vi "spotfindsettings.vi"(7 "Enum":T3(ring), 9 "already x spots found":i16, 10 "first scan?":bool, 11 "notes 2":refnum<vi>) -> (0 "settings":string, 2 "spotfinding settings":T2={"show all"=FALSE, "threshold/morph"=FALSE, "particle filter"=FALSE, "spot marks"=FALSE, "close filter"=FALSE, "connectivity 4/8"=FALSE, "range"={"Lower value"=30.0, "Upper value"=30.0}, "PSF-size"=0, "Parameters"=[]} {"range"."Upper value" format="%.2f"; "range"."Lower value" format="%.2f"; "Parameters"."Upper Value" format="%.2f"; "Parameters"."Lower Value" format="%.2f"}, 4 "coordinates":i32[][](array[numeric]))   [LabVIEW 2009]
uses:
  spotfindersettings.ctl
panel:
  in  "range":cluster{"min.":i32, "max.":i32}={"min."=30, "max."=255}
  out "Number of Particles":i32
  in  "UPDATE":bool
  in  "Selection Values":T1(array[cluster]) {"Upper Value" format="%.2f"; "Lower Value" format="%.2f"}
  in  "scroll":u32 max=1
  in  "notes":string
  in  "spot marks":bool
  in  "particle filter":bool
  in  "threshold/morph":bool
  in  "show all":bool
  in  "PSF-size":i32=15
  in  "connectivity 4/8":bool
  in  "close filter":bool
  in  "add button":bool
  in  "delete button":bool
  in  "delete element":i32 min=0 max=0
  in  "stop":bool
  # "Selection Values"
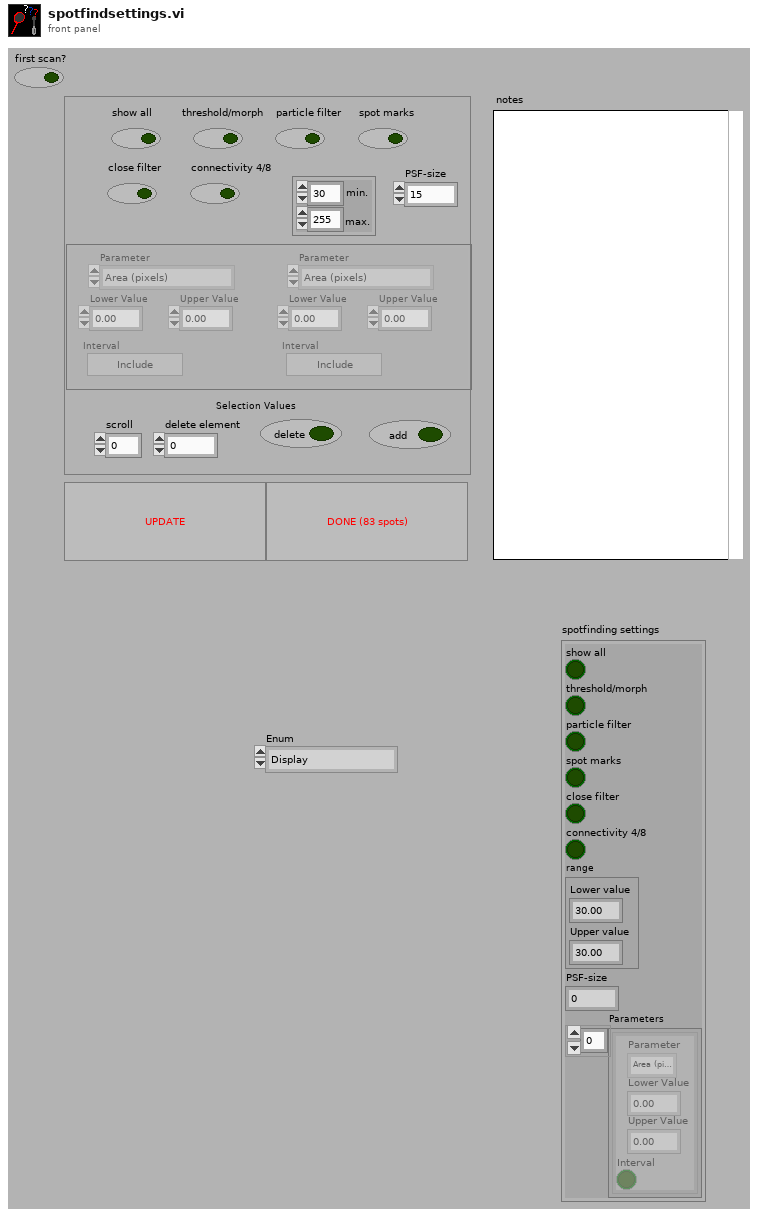
[diagram p1: front panel]
types:
  T1 = cluster{"Parameter":enum32{"Area (pixels)", "Area (calibrated)", "Number of holes", "Holes area (pixels)", "Total area (pixels)", "Scanned area (pixels)", "Ratio Area/Scanned area (%)", "Ratio Area/Total area (%)", "Center of mass (X)", "Center of mass (Y)", "Left column (X)", "Upper row (Y)", "Right column (X)", "Lower row (Y)", "Width (pixels)", "Height (pixels)", "Longest segment length", "Longest segment left column (X)", "Longest segment top row  (Y)", "Perimeter", "Holes perimeter", "SumX", "SumY", "SumXX", "SumYY", "SumXY", "Corrected projection X", "Corrected projection Y", "Moment of inertia Ixx", "Moment of inertia Iyy", "Moment of inertia Ixy", "Mean chord X", "Mean chord Y", "Max intercept", "Mean intercept perpendicular", "Particle orientation", "Equivalent ellipse minor axis", "Ellipse major axis", "Ellipse minor axis", "Ratio of equivalent ellipse axis", "Rectangle big side", "Rectangle small side", "Ratio of equivalent rectangle sides", "Elongation factor", "Compactness factor", "Heywood circularity factor", "Type factor", "Hydraulic radius", "Waddel disk diameter", "Diagonal"}, "Lower Value":sgl, "Upper Value":sgl, "Interval":bool}[]
  T2 = typedef "spotfindersettings.ctl" = cluster{"show all":bool, "threshold/morph":bool, "particle filter":bool, "spot marks":bool, "close filter":bool, "connectivity 4/8":bool, "range":cluster{"Lower value":sgl, "Upper value":sgl}, "PSF-size":i32, "Parameters":cluster{"Parameter":enum32{"Area (pixels)", "Area (calibrated)", "Number of holes", "Holes area (pixels)", "Total area (pixels)", "Scanned area (pixels)", "Ratio Area/Scanned area (%)", "Ratio Area/Total area (%)", "Center of mass (X)", "Center of mass (Y)", "Left column (X)", "Upper row (Y)", "Right column (X)", "Lower row (Y)", "Width (pixels)", "Height (pixels)", "Longest segment length", "Longest segment left column (X)", "Longest segment top row  (Y)", "Perimeter", "Holes perimeter", "SumX", "SumY", "SumXX", "SumYY", "SumXY", "Corrected projection X", "Corrected projection Y", "Moment of inertia Ixx", "Moment of inertia Iyy", "Moment of inertia Ixy", "Mean chord X", "Mean chord Y", "Max intercept", "Mean intercept perpendicular", "Particle orientation", "Equivalent ellipse minor axis", "Ellipse major axis", "Ellipse minor axis", "Ratio of equivalent ellipse axis", "Rectangle big side", "Rectangle small side", "Ratio of equivalent rectangle sides", "Elongation factor", "Compactness factor", "Heywood circularity factor", "Type factor", "Hydraulic radius", "Waddel disk diameter", "Diagonal"}, "Lower Value":sgl, "Upper Value":sgl, "Interval":bool}[]}
  T3 = enum16{"Display", "change", "get", "save", "create text", "load", "Get Refnum"}
  T4 = enum16{"Ini", "Get", "Set", "Refresh", "dump", "move", "name"}
  T5 = cluster{"show all":bool, "threshold/morph":bool, "particle filter":bool, "spot marks":bool, "close filter":bool, "connectivity 4/8":bool, "range":cluster{"Lower value":sgl, "Upper value":sgl}, "PSF-size":i32, "Parameters":cluster{"Parameter":enum32{"Area (pixels)", "Area (calibrated)", "Number of holes", "Holes area (pixels)", "Total area (pixels)", "Scanned area (pixels)", "Ratio Area/Scanned area (%)", "Ratio Area/Total area (%)", "Center of mass (X)", "Center of mass (Y)", "Left column (X)", "Upper row (Y)", "Right column (X)", "Lower row (Y)", "Width (pixels)", "Height (pixels)", "Longest segment length", "Longest segment left column (X)", "Longest segment top row  (Y)", "Perimeter", "Holes perimeter", "SumX", "SumY", "SumXX", "SumYY", "SumXY", "Corrected projection X", "Corrected projection Y", "Moment of inertia Ixx", "Moment of inertia Iyy", "Moment of inertia Ixy", "Mean chord X", "Mean chord Y", "Max intercept", "Mean intercept perpendicular", "Particle orientation", "Equivalent ellipse minor axis", "Ellipse major axis", "Ellipse minor axis", "Ratio of equivalent ellipse axis", "Rectangle big side", "Rectangle small side", "Ratio of equivalent rectangle sides", "Elongation factor", "Compactness factor", "Heywood circularity factor", "Type factor", "Hydraulic radius", "Waddel disk diameter", "Diagonal"}, "Lower Value":sgl, "Upper Value":sgl, "Interval":bool}[]}
  T6 = typedef "IMAQ Image.ctl" = refnum<image>
  T7 = enum32{"Area (pixels)", "Area (calibrated)", "Number of holes", "Holes area (pixels)", "Total area (pixels)", "Scanned area (pixels)", "Ratio Area/Scanned area (%)", "Ratio Area/Total area (%)", "Center of mass (X)", "Center of mass (Y)", "Left column (X)", "Upper row (Y)", "Right column (X)", "Lower row (Y)", "Width (pixels)", "Height (pixels)", "Longest segment length", "Longest segment left column (X)", "Longest segment top row  (Y)", "Perimeter", "Holes perimeter", "SumX", "SumY", "SumXX", "SumYY", "SumXY", "Corrected projection X", "Corrected projection Y", "Moment of inertia Ixx", "Moment of inertia Iyy", "Moment of inertia Ixy", "Mean chord X", "Mean chord Y", "Max intercept", "Mean intercept perpendicular", "Particle orientation", "Equivalent ellipse minor axis", "Ellipse major axis", "Ellipse minor axis", "Ratio of equivalent ellipse axis", "Rectangle big side", "Rectangle small side", "Ratio of equivalent rectangle sides", "Elongation factor", "Compactness factor", "Heywood circularity factor", "Type factor", "Hydraulic radius", "Waddel disk diameter", "Diagonal"}
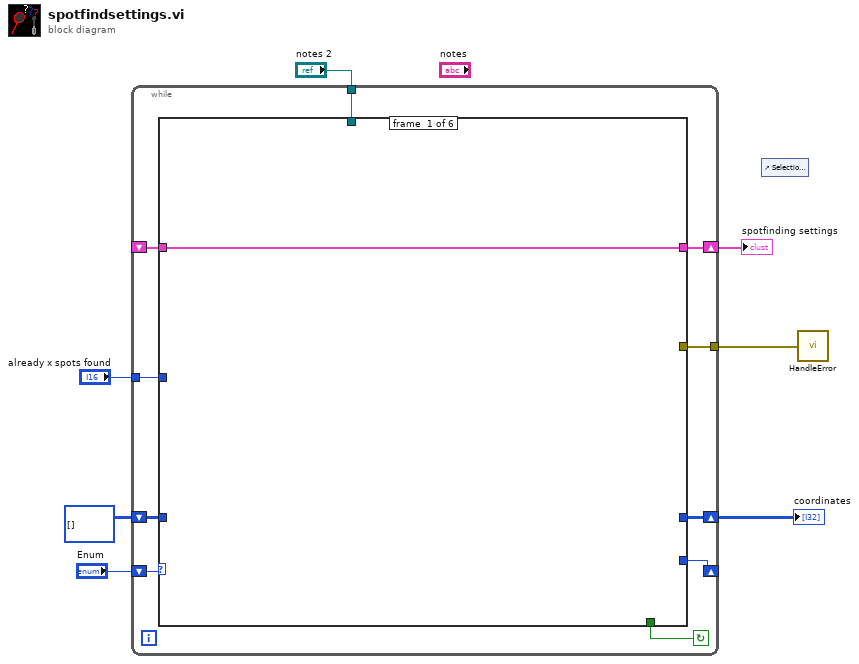
[diagram p0: block diagram]
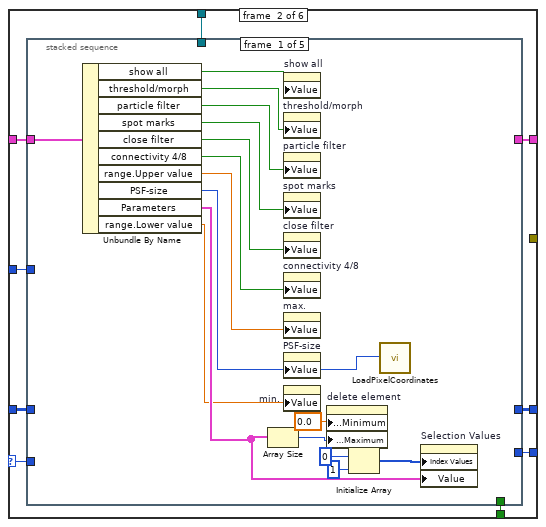
[diagram p2: hidden frame]
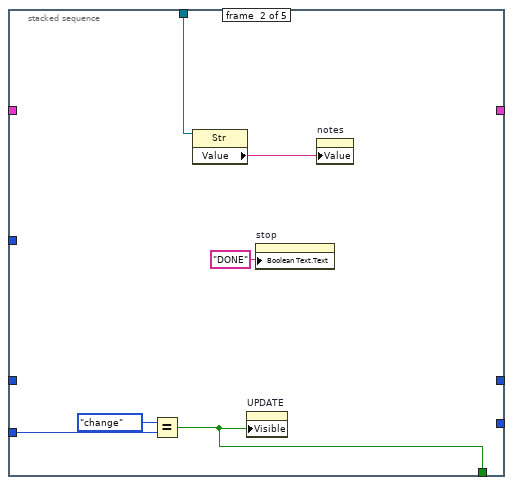
[diagram p3: hidden frame]
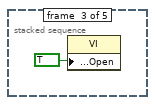
[diagram p4: hidden frame]
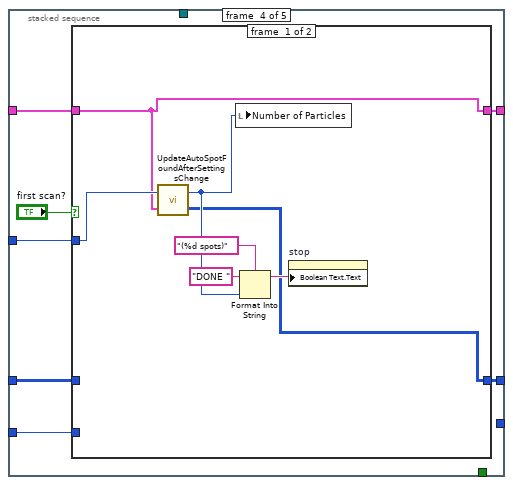
[diagram p5: hidden frame]
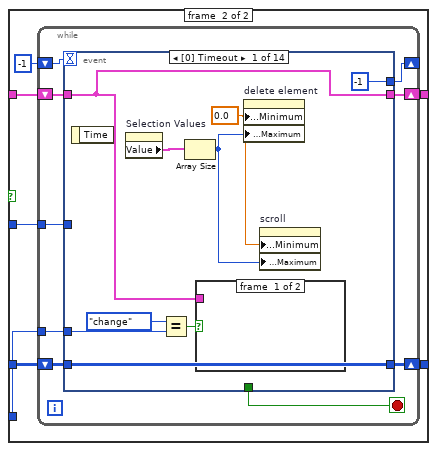
[diagram p6: hidden frame]
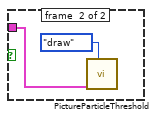
[diagram p7: hidden frame]
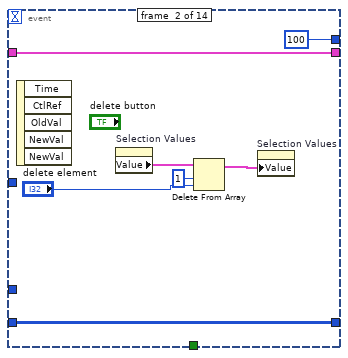
[diagram p8: hidden frame]
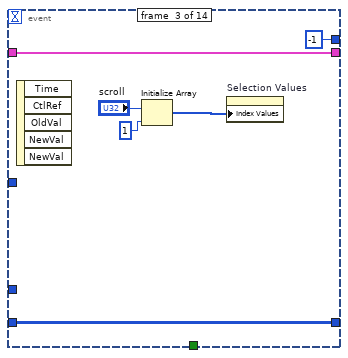
[diagram p9: hidden frame]
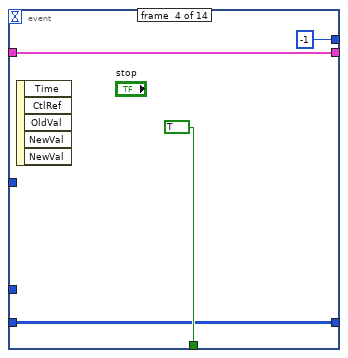
[diagram p10: hidden frame]
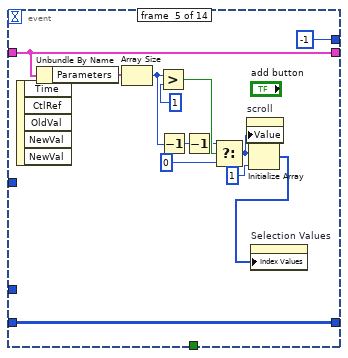
[diagram p11: hidden frame]
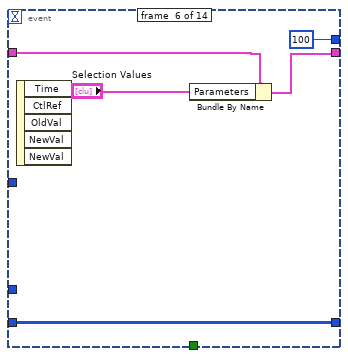
[diagram p12: hidden frame]
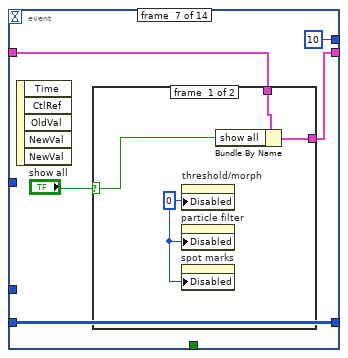
[diagram p13: hidden frame]
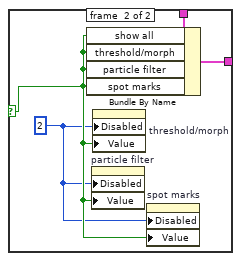
[diagram p14: hidden frame]
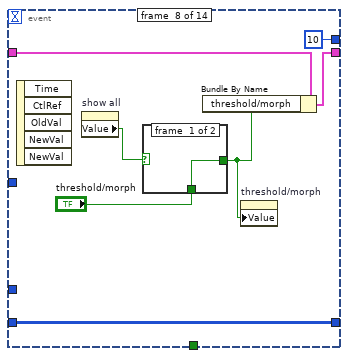
[diagram p15: hidden frame]
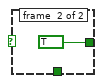
[diagram p16: hidden frame]
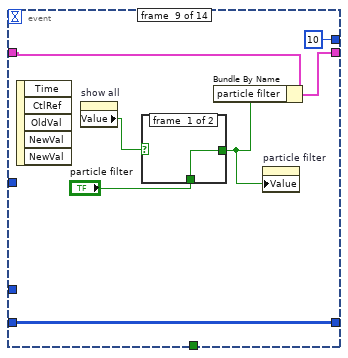
[diagram p17: hidden frame]
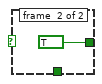
[diagram p18: hidden frame]
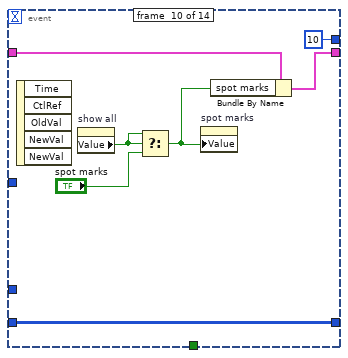
[diagram p19: hidden frame]
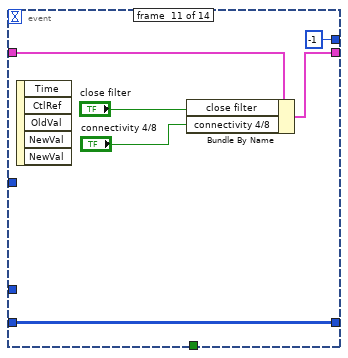
[diagram p20: hidden frame]
diagram:
  n1 = while {
    shift-right: [w8] -> w2
    shift-left: _ -> [w9]
    tunnel: [w17] -> w1
    tunnel: "notes 2" -> [w16]
    tunnel: "already x spots found" -> [w15]
    shift-right: [w12] -> _
    shift-left: "Enum" -> [w13]
    shift-right: [w10] -> w3
    shift-left: i32[][] [] ("coordinates") -> [w11]
    stop <- w14 continue-if-true
    n2 = case shown="\"Display\", \"change\"" w13 {
      selector: w13 -> [_ w21 _ _ _ _]
      tunnel: w9 -> [w18 w27 w206 w239 w245 _]
      tunnel: [_ _ _ _ w247 _] -> w17
      tunnel: w16 -> [_ w26 _ _ _ _]
      tunnel: w15 -> [_ w25 _ _ _ _]
      tunnel: [_ w24 _ _ _ _] -> w14
      tunnel: [_ w23 _ _ _ _] -> w12
      tunnel: [_ w22 w207 _ _ _] -> w10
      tunnel: w11 -> [_ w20 w207 _ _ _]
      tunnel: [w18 w19 w206 w240 w245 w252] -> w8
      frame #0 {
      }
      frame #1 {
        n3 = stacked-sequence {
          tunnel: w27 -> [w41 _ _ w57 _]
          tunnel: [_ _ _ w56 _] -> w19
          tunnel: w26 -> [_ w49 _ _ w203]
          tunnel: w25 -> [_ _ _ w55 _]
          tunnel: [_ w45 _ _ _] -> w24
          tunnel: [_ _ _ _ T3."create text" ("Enum")] -> w23
          tunnel: [_ _ _ w53 _] -> w22
          tunnel: w21 -> [_ w47 _ w54 _]
          tunnel: w20 -> [_ _ _ w52 _]
          frame #0 {
            n4 = Unbundle By Name(w41) -> ("show all"=w40:bool, "threshold/morph"=w39:bool, "particle filter"=w38:bool, "spot marks"=w37:bool, "close filter"=w36:bool, "connectivity 4/8"=w35:bool, "range.Upper value"=w34:sgl, "PSF-size"=w33:i32, "Parameters"=w29:T1, "range.Lower value"=w28:sgl)
            n5 = Array Size(array=w29) -> (size(s)=w42:i32)
            n6 = property on="show all" class="Bool (strict)"("Value"=w40) -> ()  [unwired: 2 in, 2 out]
            n7 = property on="threshold/morph" class="Bool (strict)"("Value"=w39) -> ()  [unwired: 2 in, 2 out]
            n8 = property on="particle filter" class="Bool (strict)"("Value"=w38) -> ()  [unwired: 2 in, 2 out]
            n9 = property on="spot marks" class="Bool (strict)"("Value"=w37) -> ()  [unwired: 2 in, 2 out]
            n10 = property on="close filter" class="Bool (strict)"("Value"=w36) -> ()  [unwired: 2 in, 2 out]
            n11 = property on="connectivity 4/8" class="Bool (strict)"("Value"=w35) -> ()  [unwired: 2 in, 2 out]
            n12 = property on="max." class="DigNum (strict)"("Value"=w34) -> ()  [unwired: 2 in, 2 out]
            n13 = property on="PSF-size" class="DigNum (strict)"("Value"=w33) -> ()  [unwired: 2 in, 2 out]
            n14 = property on="min." class="DigNum (strict)"("Value"=w28) -> ()  [unwired: 2 in, 2 out]
            n15 = property on="delete element" class="Digital (strict)"("Data Entry Limits:Minimum"=0.0 ("Data Range:Minimum"), "Data Entry Limits:Maximum"=w42) -> ()  [unwired: 2 in, 2 out]
            n16 = Initialize Array(u32 0 ("element"), 1 ("dimension size")) -> (w30:u32[])
            n17 = call "LoadPixelCoordinates.vi"("spotsize (radius pixel)"=w33) -> ()
            n18 = property on="Selection Values" class="Array (strict)"("Index Values"=w30, "Value"=w29) -> ()  [unwired: 2 in, 2 out]
          }
          frame #1 {
            n19 = Equal?(x=T3."change", y=w47) -> (x = y?=w45:bool)
            n20 = property class="Str"(reference=w49) -> ("Value"=w48:string)  [unwired: 1 in, 2 out]
            n21 = property on="UPDATE" class="Bool"("Visible"=w45) -> ()  [unwired: 2 in, 2 out]
            n22 = property on="stop" class="Bool"("Boolean Text.Text"="DONE") -> ()  [unwired: 2 in, 2 out]
            n23 = property on="notes" class="String"("Value"=w48) -> ()  [unwired: 2 in, 2 out]
          }
          frame #2 {
            n24 = property class="VI"("Front Panel Window:Open"=TRUE) -> ()  [unwired: 2 in, 2 out]
          }
          frame #3 {
            n25 = case shown="True" "first scan?" {
              tunnel: w57 -> [w58 w70]
              tunnel: [w58 w69] -> w56
              tunnel: w55 -> [w59 w68]
              tunnel: w54 -> [_ w67]
              tunnel: [w60 w66] -> w53
              tunnel: w52 -> [_ w65]
              frame #0 {
                n26 = call "UpdateAutoSpotFoundAfterSettingsChange.vi"("spotfinding settings"=w58, "already x spots found"=w59) -> ("coordinates"=w60:i32[][], "Number of Particles"=w61:i32)
                n27 = local write "Number of Particles"(w61) -> ()
                n28 = Format Into String(format string="(%d spots)", initial string="DONE ", w61) -> (resulting string=w64:string)  [unwired: 1 in, 1 out]
                n29 = property on="stop" class="Bool"("Boolean Text.Text"=w64) -> ()  [unwired: 2 in, 2 out]
              }
              frame #1 {
                n30 = while {
                  shift-right: [w78] -> _
                  shift-left: -1 -> [w79]
                  shift-right: [w76] -> w69
                  shift-left: w70 -> [w77]
                  tunnel: w68 -> [w75]
                  tunnel: w67 -> [w74]
                  shift-right: [w73] -> w66
                  shift-left: w65 -> [w72]
                  stop <- w80 stop-if-true
                  n31 = event shown="[0] Timeout" {
                    selector: _ -> [_ _ _ _ _ _ _ _ _ _ _ _ _ _]
                    dyn-events: _ -> [_ _ _ _ _ _ _ _ _ _ _ _ _ _]
                    timeout: w79 -> [_ _ _ _ _ _ _ _ _ _ _ _ _ _]
                    tunnel: [_ _ _ TRUE _ _ _ _ _ _ _ _ _ TRUE] -> w80
                    tunnel: [-1 100 -1 -1 -1 100 10 10 10 10 -1 -1 -1 _] -> w78
                    tunnel: w77 -> [w82 w95 w104 w106 w120 w123 w129 w146 w151 w164 w170 w183 w184 w193]
                    tunnel: [w82 w95 w104 w106 w120 w122 w128 w145 w152 w163 w169 w182 w184 w193] -> w76
                    tunnel: w75 -> [_ _ _ _ _ _ _ _ _ _ _ _ w190 _]
                    tunnel: [w81 w92 w99 w105 w109 w124 w127 w140 w149 w161 w165 w179 w189 w192] -> w73
                    tunnel: w74 -> [w84 _ _ _ _ _ _ _ _ _ _ _ _ _]
                    tunnel: w72 -> [w81 w92 w99 w105 w109 w124 w127 w140 w149 w161 w165 w179 _ w192]
                    event #0 {
                      w87 = 0.0 ("Data Range:Minimum")
                      n32 = event-data() -> ()  [unwired: 1 in, 1 out]
                      n33 = property on="Selection Values" class="Array (strict)"() -> ("Value"=w86:T1)  [unwired: 2 in, 2 out]
                      n34 = Equal?(x=T3."change", y=w84) -> (x = y?=w85:bool)
                      n35 = Array Size(array=w86) -> (size(s)=w88:i32)
                      n36 = case shown="True" w85 {
                        tunnel: w82 -> [_ w90]
                        frame #0 {
                        }
                        frame #1 {
                          n37 = call "PictureParticleThreshold.vi"("Enum"=enum16{"new", "input", "draw", "dump"}."draw", "spotfinding settings"=w90) -> ()  [unwired: 6 in, 2 out]
                        }
                      }
                      n38 = property on="delete element" class="Digital (strict)"("Data Entry Limits:Minimum"=w87, "Data Entry Limits:Maximum"=w88) -> ()  [unwired: 2 in, 2 out]
                      n39 = property on="scroll" class="DigNum (strict)"("Data Entry Limits:Minimum"=w87, "Data Entry Limits:Maximum"=w88) -> ()  [unwired: 2 in, 2 out]
                    }
                    event #1 {
                      n40 = event-data() -> ()  [unwired: 1 in, 5 out]
                      n41 = property on="Selection Values" class="Array (strict)"() -> ("Value"=w93:T1)  [unwired: 2 in, 2 out]
                      n42 = Delete From Array(array=w93, length=1, index="delete element") -> (array with subset deleted=w94:T1)  [unwired: 1 out]
                      n43 = property on="Selection Values" class="Array (strict)"("Value"=w94) -> ()  [unwired: 2 in, 2 out]
                    }
                    event #2 {
                      n44 = event-data() -> ()  [unwired: 1 in, 5 out]
                      n45 = Initialize Array("scroll", 1 ("dimension size")) -> (w100:u32[])
                      n46 = property on="Selection Values" class="Array (strict)"("Index Values"=w100) -> ()  [unwired: 2 in, 2 out]
                    }
                    event #3 {
                      n47 = event-data() -> ()  [unwired: 1 in, 5 out]
                    }
                    event #4 {
                      n48 = event-data() -> ()  [unwired: 1 in, 5 out]
                      n49 = Unbundle By Name(w120) -> ("Parameters"=w119:T1)
                      n50 = Array Size(array=w119) -> (size(s)=w115:i32)
                      n51 = Greater?(x=w115, y=1) -> (0:w117:bool)
                      n52 = Decrement(x=w115) -> (x-1=w114:i32)
                      n53 = Decrement(x=w114) -> (x-1=w113:i32)
                      n54 = Select(t=w113, s=w117, f=u32 0) -> (s? t:f=w111:u32)
                      n55 = property on="scroll" class="DigNum (strict)"("Value"=w111) -> ()  [unwired: 2 in, 2 out]
                      n56 = Initialize Array(w111, 1 ("dimension size")) -> (w110:u32[])
                      n57 = property on="Selection Values" class="Array (strict)"("Index Values"=w110) -> ()  [unwired: 2 in, 2 out]
                    }
                    event #5 {
                      n58 = event-data() -> ()  [unwired: 1 in, 5 out]
                      n59 = Bundle By Name(cluster=w123, "Parameters"="Selection Values") -> (w122:T5)
                    }
                    event #6 {
                      n60 = event-data() -> ()  [unwired: 1 in, 5 out]
                      n61 = case shown="True" "show all" {
                        selector: "show all" -> [w133 w137]
                        tunnel: w129 -> [w135 w139]
                        tunnel: [w134 w138] -> w128
                        frame #0 {
                          w132 = u8 0 ("Disabled")
                          n62 = property on="threshold/morph" class="Bool (strict)"("Disabled"=w132) -> ()  [unwired: 2 in, 2 out]
                          n63 = property on="particle filter" class="Bool (strict)"("Disabled"=w132) -> ()  [unwired: 2 in, 2 out]
                          n64 = property on="spot marks" class="Bool (strict)"("Disabled"=w132) -> ()  [unwired: 2 in, 2 out]
                          n65 = Bundle By Name(cluster=w135, "show all"=w133) -> (w134:T5)
                        }
                        frame #1 {
                          w136 = 2
                          n66 = Bundle By Name(cluster=w139, "show all"=w137, "threshold/morph"=w137, "particle filter"=w137, "spot marks"=w137) -> (w138:T5)
                          n67 = property on="particle filter" class="Bool (strict)"("Disabled"=w136, "Value"=w137) -> ()  [unwired: 2 in, 2 out]
                          n68 = property on="threshold/morph" class="Bool (strict)"("Disabled"=w136, "Value"=w137) -> ()  [unwired: 2 in, 2 out]
                          n69 = property on="spot marks" class="Bool (strict)"("Disabled"=w136, "Value"=w137) -> ()  [unwired: 2 in, 2 out]
                        }
                      }
                    }
                    event #7 {
                      n70 = event-data() -> ()  [unwired: 1 in, 5 out]
                      n71 = property on="show all" class="Boolean (strict)"() -> ("Value"=w144:bool)  [unwired: 2 in, 2 out]
                      n72 = case shown="True" w144 {
                        tunnel: [w147 TRUE] -> w142
                        tunnel: "threshold/morph" -> [w147 _]
                        frame #0 {
                        }
                        frame #1 {
                        }
                      }
                      n73 = Bundle By Name(cluster=w146, "threshold/morph"=w142) -> (w145:T5)
                      n74 = property on="threshold/morph" class="Boolean (strict)"("Value"=w142) -> ()  [unwired: 2 in, 2 out]
                    }
                    event #8 {
                      n75 = event-data() -> ()  [unwired: 1 in, 5 out]
                      n76 = property on="show all" class="Boolean (strict)"() -> ("Value"=w155:bool)  [unwired: 2 in, 2 out]
                      n77 = case shown="True" w155 {
                        tunnel: [w156 TRUE] -> w153
                        tunnel: "particle filter" -> [w156 _]
                        frame #0 {
                        }
                        frame #1 {
                        }
                      }
                      n78 = Bundle By Name(cluster=w151, "particle filter"=w153) -> (w152:T5)
                      n79 = property on="particle filter" class="Boolean (strict)"("Value"=w153) -> ()  [unwired: 2 in, 2 out]
                    }
                    event #9 {
                      n80 = event-data() -> ()  [unwired: 1 in, 5 out]
                      n81 = property on="show all" class="Boolean (strict)"() -> ("Value"=w160:bool)  [unwired: 2 in, 2 out]
                      n82 = Select(t=w160, s=w160, f="spot marks") -> (s? t:f=w158:bool)
                      n83 = property on="spot marks" class="Bool (strict)"("Value"=w158) -> ()  [unwired: 2 in, 2 out]
                      n84 = Bundle By Name(cluster=w164, "spot marks"=w158) -> (w163:T5)
                    }
                    event #10 {
                      n85 = event-data() -> ()  [unwired: 1 in, 5 out]
                      n86 = Bundle By Name(cluster=w170, "close filter"="close filter", "connectivity 4/8"="connectivity 4/8") -> (w169:T5)
                    }
                    event #11 {
                      n87 = event-data() -> ()  [unwired: 1 in, 5 out]
                      n88 = Unbundle By Name("range") -> ("min."=w176:i32, "max."=w175:i32)
                      n89 = Max & Min(x=w176, y=w175) -> (max(x,y)=w173:i32, min(x,y)=w172:i32)
                      n90 = Bundle By Name(cluster="range", "max."=w173, "min."=w172) -> (w171:cluster{"min.":i32, "max.":i32})
                      n91 = Bundle(cluster=cluster{"Lower value":sgl, "Upper value":sgl} {"Lower value"=128.0, "Upper value"=255.0} ("Range"), "Lower value"=w172, "Upper value"=w173) -> (w178:cluster{"Lower value":sgl, "Upper value":sgl})
                      n92 = Bundle By Name(cluster=w183, "range"=w178, "PSF-size"="PSF-size") -> (w182:T5)
                      n93 = property on="range" class="Cluster (strict)"("Value"=w171) -> ()  [unwired: 2 in, 2 out]
                      n94 = call "LoadPixelCoordinates.vi"("spotsize (radius pixel)"="PSF-size") -> ()
                    }
                    event #12 {
                      n95 = event-data() -> ()  [unwired: 1 in, 5 out]
                      n96 = call "UpdateAutoSpotFoundAfterSettingsChange.vi"("spotfinding settings"=w184, "already x spots found"=w190) -> ("coordinates"=w189:i32[][], "Number of Particles"=w187:i32)
                      "Number of Particles" <- w187
                      n97 = Format Into String(format string="(%d spots)", initial string="DONE ", w187) -> (resulting string=w188:string)  [unwired: 1 in, 1 out]
                      n98 = property on="stop" class="Bool"("Boolean Text.Text"=w188) -> ()  [unwired: 2 in, 2 out]
                    }
                    event #13 {
                      n99 = event-data() -> ()  [unwired: 1 in, 3 out]
                      n100 = event-data("Discard?"=FALSE) -> ()  [unwired: 1 in, 1 out]
                    }
                  }
                }
              }
            }
          }
          frame #4 {
            n101 = call "FilePathGlobal.vi"("set?"=FALSE) -> ("Image Path 2"=w198:path)  [unwired: 1 in, 2 out]
            n102 = property on="notes" class="Str"() -> ("Value"=w204:string)  [unwired: 2 in, 2 out]
            n103 = property class="VI"("Front Panel Window:Open"=FALSE) -> ()  [unwired: 2 in, 2 out]
            n104 = call "Intensityduplex.vi"("Enum"=T4."Get") -> ("Image Duplicate (out)"=w200:T6)  [unwired: 4 in, 1 out]
            n105 = call "changefilename.vi"("suffix"="_spots.png", "path in"=w198) -> ("path out"=w196:path)  [unwired: 1 out]
            n106 = property on="Property Node" class="Str"(reference=w203, "Value"=w204) -> ()  [unwired: 1 in, 2 out]
            n107 = call-poly "IMAQ Write File 2"("File Path"=w196, "Image"=w200) -> ()  [unwired: 8 in, 2 out]
          }
        }
      }
      frame #2 {
        n108 = stacked-sequence {
          seq-local: [w214 _] -> [_ w229]
          tunnel: w206 -> [w218 w227]
          frame #0 {
            n109 = Unbundle By Name(w218) -> ("close filter"=w217:bool, "connectivity 4/8"=w216:bool, "range.Lower value"=w215:sgl, "range.Upper value"=w208:sgl)
            n110 = Format Into String(format string="%s %s\\n%s %s\\n%s %d\\n%s %d\\n", "close filter: ", w217, "connectivity 4/8:" ("input 3"), w216, "threshold (min): ", w215, "threshold (max): ", w208) -> (resulting string=w213:string)  [unwired: 2 in, 1 out]
            n111 = property on="Number of Particles" class="Digital (strict)"() -> ("Value"=w212:i32)  [unwired: 2 in, 2 out]
            n112 = Format Into String(format string="\\n%d\\sspot(s)\\sfound\\n", w212) -> (resulting string=w211:string)  [unwired: 2 in, 1 out]
            n113 = Concatenate Strings(w211, w213) -> (w214:string)
          }
          frame #1 {
            n114 = Unbundle By Name(w227) -> ("Parameters"=w223:T1)
            n115 = for {
              shift-right: [w236] -> w226
              shift-left: "" -> [w237]
              tunnel: w223 -> [w234] mode=indexing
              n116 = Unbundle By Name(w234) -> ("Parameter"=w233:T7, "Lower Value"=w232:sgl, "Upper Value"=w231:sgl, "Interval"=w230:bool)
              n117 = Format Into String(format string="Parameter: %s\\n\\t lower value: %.2f\\n\\t upper value: %.2f\\n\\t include: %s\\n", w233, w232, w231, w230) -> (resulting string=w238:string)  [unwired: 2 in, 1 out]
              n118 = Concatenate Strings(w237, w238) -> (w236:string)
            }
            n119 = Concatenate Strings(w229, "selection values:\n", w226) -> (→"settings":string)
          }
        }
      }
      frame #3 {
        n120 = Current VI's Path() -> (path=w244:path)
        n121 = Strip Path(path=w244) -> (stripped path=w243:path)  [unwired: 1 out]
        n122 = Build Path(base path=w243, name or relative path="autospotting.set") -> (appended path=w241:path)
        n123 = Read from Binary File(5:w239, 11:w241) -> (2:w240:T5)  [unwired: 4 in, 3 out]
      }
      frame #4 {
        n124 = Current VI's Path() -> (path=w251:path)
        n125 = Strip Path(path=w251) -> (stripped path=w250:path)  [unwired: 1 out]
        n126 = Build Path(base path=w250, name or relative path="autospotting.set") -> (appended path=w248:path)
        n127 = Write to Binary File(file (use dialog)=w248, data=w245, 5:TRUE ("prepend array or string size? (T)")) -> (error out=w247:errorcluster)  [unwired: 3 in, 2 out]
      }
      frame #5 {
        n128 = property on="spotfinding settings" class="Clust (strict)"() -> ("Value"=w252:T5)  [unwired: 2 in, 2 out]
      }
    }
  }
  "spotfinding settings" <- w2
  "coordinates" <- w3
  n129 = control-ref of="Selection Values"() -> ()  [unwired: 1 out]
  n130 = call "HandleError.vi"("error in (no error)"=w1) -> ()
